vi "index_one_axis.vi"(8 "x_index":i32, 9 "curve_sel":i32, 11 "graph_data":cluster{"array type (2D Dbl)":dbl[], dbl[]}[](array[cluster])) -> (2 "Y":dbl, 3 "X":dbl)   [LabVIEW 2025]
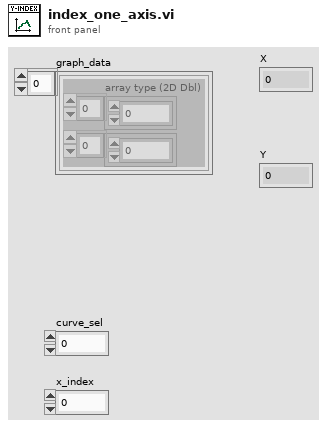
[diagram p1: front panel]
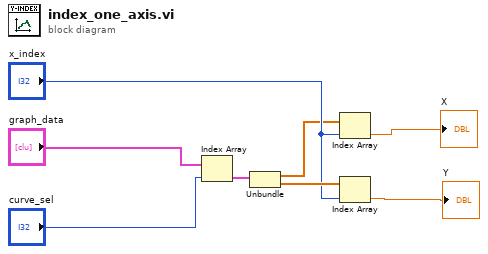
[diagram p0: block diagram]
diagram:
  n1 = Index Array(array="graph_data", index="curve_sel") -> (element=w6:cluster{"array type (2D Dbl)":dbl[], dbl[]})
  n2 = Unbundle(w6) -> ("array type (2D Dbl)"=w4:dbl[], w7:dbl[])
  n3 = Index Array(array=w4, index="x_index") -> (element=→"X":dbl)
  n4 = Index Array(array=w7, index="x_index") -> (element=→"Y":dbl)
